vi "Zeta of Positive Number.vi"(10 "x":cdb=1.0+0.0i) -> (3 "z(x)":cdb format="%#_20g")   [LabVIEW 2017, in "NI_Gmath.lvlib"]
uses:
  <vilib>/gmath/NI_Gmath.lvlib
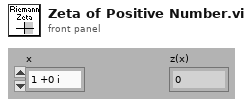
[diagram p1: front panel]
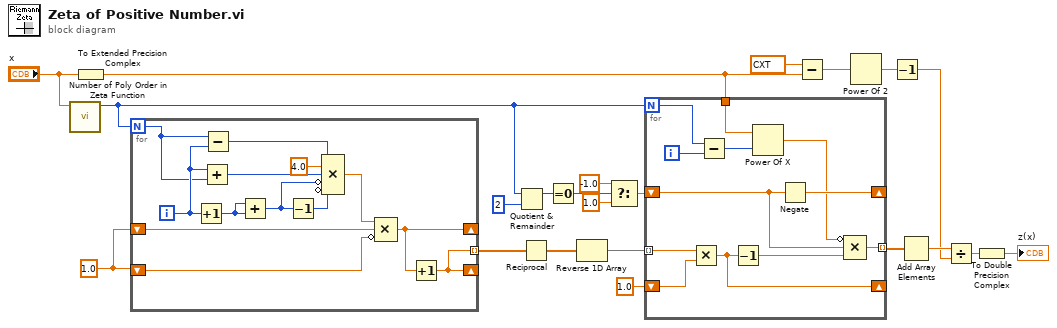
[diagram p0: block diagram]
diagram:
  w5 = 1.0 ("n 2")
  n1 = call <vilib>:"Number of Poly Order in Zeta Function.vi"("x"="x") -> ("n"=w3:i32)  [unwired: 10 out]
  n2 = To Extended Precision Complex(1:"x") -> (0:w2:cxt)
  n3 = for {
    N: w3 -> [w27]
    shift-right: [w26] -> _
    shift-left: w5 -> [w25]
    shift-right: [w28] -> _
    shift-left: w5 -> [w24]
    tunnel: [w26] -> w12 mode=indexing
    i -> [w30]
    n4 = Increment(x=w30) -> (x+1=w33:i32)
    n5 = Add(x=w30, y=w27) -> (x+y=w35:i32)
    n6 = Subtract(x=w27, y=w30) -> (x-y=w23:i32)
    n7 = Add(x=w33, y=w33) -> (x+y=w32:i32)
    n8 = Decrement(x=w32) -> (x-1=w31:i32)
    n9 = Compound Arithmetic op=MULTIPLY(w23, 4.0 ("n 2"), w35, invert w32, invert w31) -> (w29:dbl)
    n10 = Compound Arithmetic op=MULTIPLY(w29, w24, invert w25) -> (w28:dbl)
    n11 = Increment(x=w28) -> (x+1=w26:dbl)
  }
  n12 = Quotient & Remainder(x=w3, y=2) -> (x-y*floor(x/y)=w10:i32)  [unwired: 1 out]
  n13 = Reciprocal(x=w12) -> (1/x=w20:dbl[])
  n14 = Equal To 0?(x=w10) -> (x = 0?=w9:bool)
  n15 = Reverse 1D Array(array=w20) -> (reversed array=w22:dbl[])
  n16 = Select(t=-1.0, s=w9, f=1.0) -> (s? t:f=w8:dbl)
  n17 = for {
    N: w3 -> [w40]
    tunnel: w22 -> [w47] mode=indexing
    shift-right: [w45] -> _
    shift-left: 1.0 ("element") -> [w46]
    shift-right: [w44] -> _
    shift-left: w8 -> [w43]
    tunnel: [w37] -> w17 mode=indexing
    tunnel: w2 -> [w36]
    i -> [w41]
    n18 = Multiply(x=w47, y=w46) -> (x*y=w45:dbl)
    n19 = Subtract(x=w40, y=w41) -> (x-y=w39:i32)
    n20 = Decrement(x=w45) -> (x-1=w42:dbl)
    n21 = Power Of X(1:w39, 2:w36) -> (0:w38:cxt)
    n22 = Negate(x=w43) -> (-x=w44:dbl)
    n23 = Compound Arithmetic op=MULTIPLY(invert w38, w43, w42) -> (w37:cxt)
  }
  n24 = Subtract(x=cxt 1.0+0.0i, y=w2) -> (x-y=w18:cxt)
  n25 = Power Of 2(x=w18) -> (2^x=w16:cxt)
  n26 = Decrement(x=w16) -> (x-1=w14:cxt)
  n27 = Add Array Elements(numeric array=w17) -> (sum=w15:cxt)
  n28 = Divide(x=w15, y=w14) -> (x/y=w13:cxt)
  n29 = To Double Precision Complex(1:w13) -> (0:→"z(x)":cdb)
